vi "MakeCurInfo.vi"() -> ()   [LabVIEW 2012, in "WaveGraphX.xctl"]
doc: "制作图例的答题信息,其输出图片可作为游标图列模板"
uses:
  WaveGraphX.xctl
panel:
  in  "DemoOut":picture
  out "Picture Out":picture
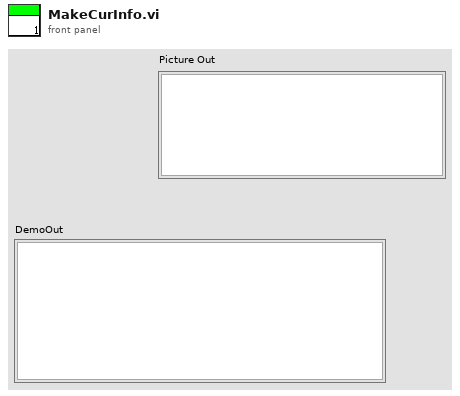
[diagram p1: front panel]
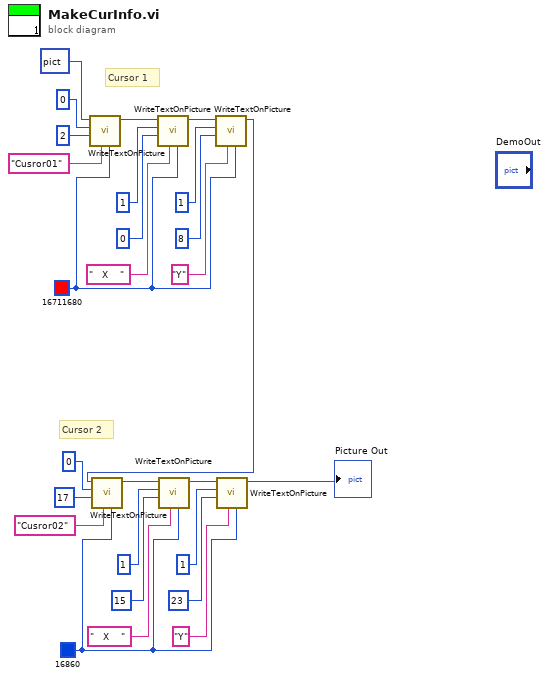
[diagram p0: block diagram]
diagram:
  w4 = u32 16860 ("颜色")
  w3 = u32 16711680 ("颜色")
  # "Cursor 1"
  # "Cursor 2"
  n1 = call "WriteTextOnPicture.vi"("颜色"=w3, "文本"="Cusror01", "列索引"=u32 2, "行索引"=u32 0, "Origin Picture"=picture data[5B]) -> ("Picture Out"=w23:picture)  [unwired: 6 in]
  n2 = call "WriteTextOnPicture.vi"("颜色"=w3, "文本"="   X    ", "列索引"=u32 0, "行索引"=u32 1, "Origin Picture"=w23) -> ("Picture Out"=w16:picture)  [unwired: 6 in]
  n3 = call "WriteTextOnPicture.vi"("颜色"=w3, "文本"="Y", "列索引"=u32 8, "行索引"=u32 1, "Origin Picture"=w16) -> ("Picture Out"=w2:picture)  [unwired: 6 in]
  n4 = call "WriteTextOnPicture.vi"("颜色"=w4, "文本"="Cusror02", "列索引"=u32 17, "行索引"=u32 0, "Origin Picture"=w2) -> ("Picture Out"=w8:picture)  [unwired: 6 in]
  n5 = call "WriteTextOnPicture.vi"("颜色"=w4, "文本"="   X    ", "列索引"=u32 15, "行索引"=u32 1, "Origin Picture"=w8) -> ("Picture Out"=w15:picture)  [unwired: 6 in]
  n6 = call "WriteTextOnPicture.vi"("颜色"=w4, "文本"="Y", "列索引"=u32 23, "行索引"=u32 1, "Origin Picture"=w15) -> ("Picture Out"=→"Picture Out":picture)  [unwired: 6 in]
